vi "Inlet Convert Temp to Volt LCP3.vi"(1 "Inlet Temperature":dbl) -> (0 "Inlet Voltage":dbl)   [LabVIEW 2014]
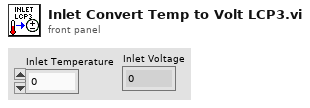
[diagram p1: front panel]
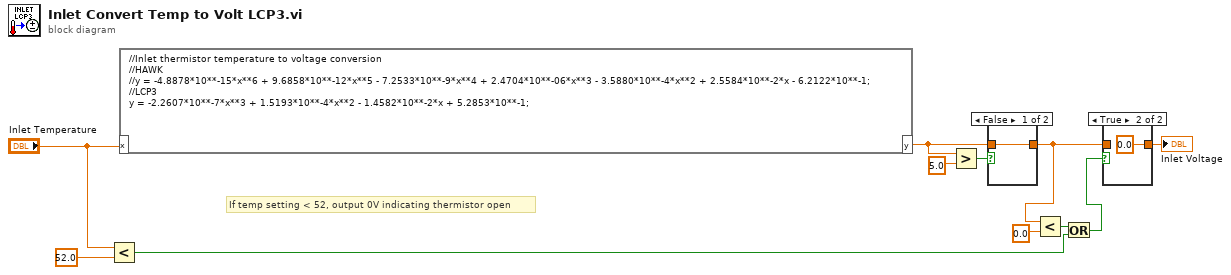
[diagram p0: block diagram]
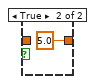
[diagram p3: hidden frame]
diagram:
  # "If temp setting < 52, output 0V indicating thermistor open"
  n1 = Less?(x="Inlet Temperature", y=52.0) -> (x < y?=w1:bool)
  n2 = formula code="//Inlet thermistor temperature to voltage conversion\n//HAWK\n//y = -4.8878*10**-15*x**6 + 9.6858*10**-12*x**5 - 7.2533*10**-9*x**4 + 2.4704*10**-06*x**3 - 3.5880*10**-4*x**2 + 2.5584*10**-2*x - 6.2122*10**-1;\n//LCP3\ny = -2.2607*10**-7*x**3 + 1.5193*10**-4*x**2 - 1.4582*10**-2*x + 5.2853*10**-1;"("x"="Inlet Temperature") -> ("y"=w10:dbl)
  n3 = Greater?(x=w10, y=5.0) -> (0:w8:bool)
  n4 = case shown="False" w8 {
    tunnel: [w12 5.0 ("y")] -> w6
    tunnel: w10 -> [w12 _]
    frame False {
    }
    frame True {
    }
  }
  n5 = Less?(x=w6, y=0.0) -> (x < y?=w5:bool)
  n6 = Or(x=w5, y=w1) -> (x .or. y?=w4:bool)
  n7 = case shown="True" w4 {
    tunnel: [w14 0.0 ("y")] -> w7
    tunnel: w6 -> [w14 _]
    frame False {
    }
    frame True {
    }
  }
  "Inlet Voltage" <- w7
